vi "optagefrekvenssignal0.4.vi"() -> ()   [LabVIEW 2014]
uses:
  <vilib>/measure/maspectr.llb/FFT Power Spectrum and PSD for 1 Chan.vi
  <vilib>/measure/NI_MAPro.lvlib
panel:
  out "Maks frekvens":dbl
  out "FFT af lydsignal":dbl[](graph)
  out "Lydsignal":waveform(dbl)(graph)
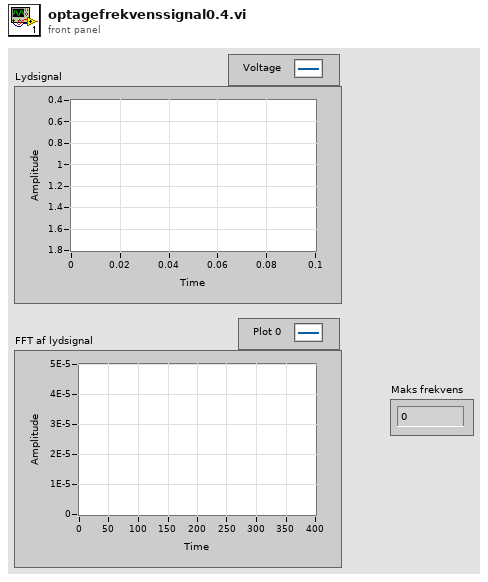
[diagram p1: front panel]
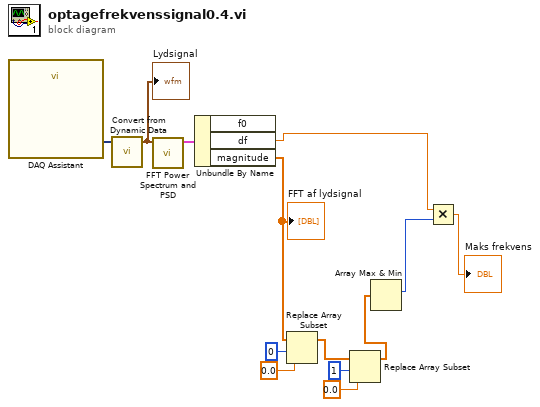
[diagram p0: block diagram]
diagram:
  n1 = call "DAQ Assistant"() -> ("data"=w13:dynamicdata)  [unwired: 17 in, 2 out]
  n2 = call "Convert from Dynamic Data"("Dynamic Data Type"=w13) -> ("Waveform"=w12:waveform(dbl))  [unwired: 3 in]
  "Lydsignal" <- w12
  n3 = call-poly <vilib>:"FFT Power Spectrum and PSD.vi"("time signal"=w12) -> ("Power Spectrum / PSD"=w11:cluster{"f0":dbl, "df":dbl, "magnitude":dbl[]})  [unwired: 7 in, 3 out]
  n4 = Unbundle By Name(w11) -> ("df"=w2:dbl, "magnitude"=w8:dbl[])  [unwired: 1 out]
  "FFT af lydsignal" <- w8
  n5 = Replace Array Subset(array=w8, new element=0.0 ("new element/subarray"), index=0) -> (w7:dbl[])
  n6 = Replace Array Subset(array=w7, new element=0.0 ("new element/subarray"), index=1) -> (w4:dbl[])
  n7 = Array Max & Min(array=w4) -> (max index (indices)=w3:i32)  [unwired: 3 out]
  n8 = Multiply(x=w2, y=w3) -> (x*y=→"Maks frekvens":dbl)
